vi "Close Document.vi"(8 "error in (no error)":errorcluster, 11 "Document API in":refnum<class "Document API.lvclass">) -> (0 "error out":errorcluster, 3 "Document Path":path)   [LabVIEW 2017, in "Document API.lvlib" / "Document API.lvclass"]
doc: "Saves the <b>Document in</b> to the <b>Document Path</b> location given in the create or open method and closes the underlying <b>Document in</b> resources, from which the Document was created. \n\nNotes:\n - If <b>Document Path</b> location given in the create or open method is empty or is <Not A Path> or is a directory, the VI saves the document at a generated file path into the temporary directory. \n - Once this has been called, no further operations, updates or reads should be performed on the <b>Document</b>."
uses:
  Document API.lvclass
  Document API.lvclass/Document API.ctl
  NPOI_Document/npoiDocument/npoiDocument.lvclass/npoiDocument.ctl
  NPOI_Document/npoiDocument/Get Document.Path.vi
  NPOI_Document/npoiDocument/npoiDocument.lvclass
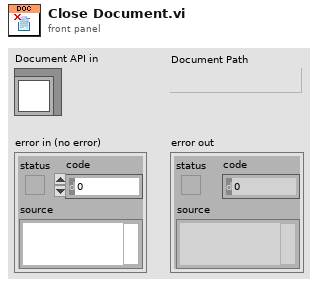
[diagram p1: front panel]
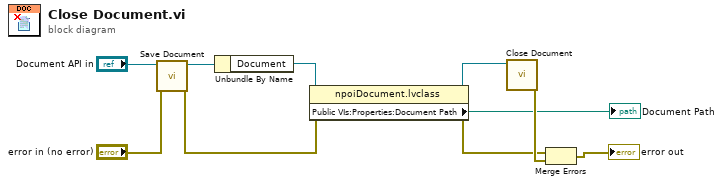
[diagram p0: block diagram]
diagram:
  n1 = call "Save Document.vi"("error in (no error)"="error in (no error)", "Document API in"="Document API in") -> ("error out"=w4:errorcluster, "Document API out"=w1:refnum<class "Document API.lvclass">)  [unwired: 8 in]
  n2 = Unbundle By Name(w1) -> ("Document"=w10:refnum<class "npoiDocument.lvclass">)
  n3 = property class="npoiDocument.lvclass"(reference=w10, error in=w4) -> (reference out=w7:refnum<class "npoiDocument.lvclass">, error out=w5:errorcluster, "Public VIs:Properties:Document Path"=→"Document Path":path)
  n4 = call "Close Document.vi"("Document in"=w7) -> ("error out"=w8:errorcluster)  [unwired: 10 in]
  n5 = Merge Errors(w5, w8) -> (→"error out":errorcluster)
